vi "predict.vi"(8 "error in (no error)":errorcluster caption="entrée d'erreur (pas d'erreur)", 11 "IsotonicRegression.lvclass 2":refnum<class "IsotonicRegression.lvclass">) -> (0 "error out":errorcluster caption="sortie d'erreur", 2 "C":dbl[][](array[numeric]), 3 "IsotonicRegression.lvclass":refnum<class "IsotonicRegression.lvclass">)   [LabVIEW 2020, in "IsotonicRegression.lvclass"]
doc: "Predict new data by linear interpolation."
uses:
  IsotonicRegression.lvclass
  C:/Users/cipop/TDF Dropbox/2_Technologies de France/1 - Services et Etudes/PLAIY/2 - DEV/PLAIYLAB/code/Python/Python.lvclass
  C:/Users/cipop/TDF Dropbox/2_Technologies de France/1 - Services et Etudes/PLAIY/2 - DEV/PLAIYLAB/code/Model/Model.lvclass
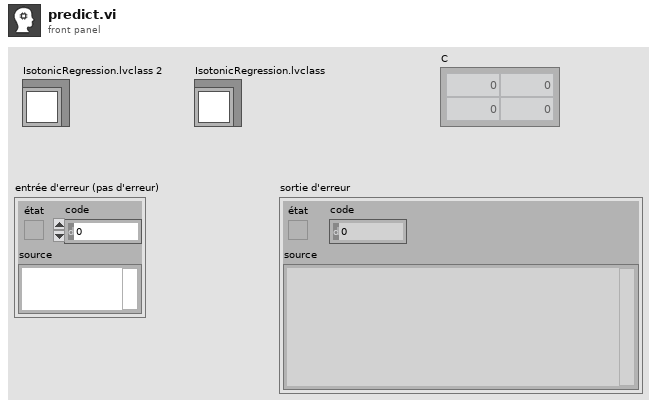
[diagram p1: front panel]
types:
  T1 = typedef "data.ctl" = cluster{"name":string, "X":dbl[][]}
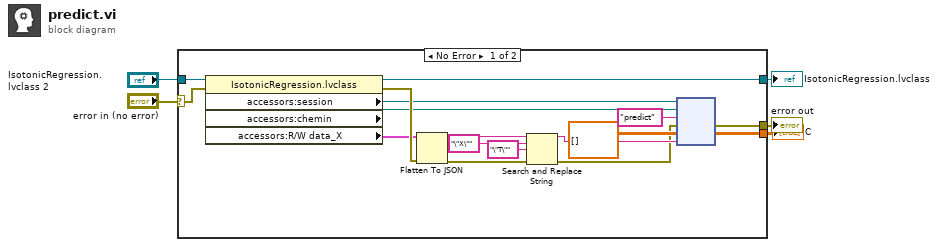
[diagram p0: block diagram]
diagram:
  n1 = case shown="No Error" "error in (no error)" {
    selector: "error in (no error)" -> [w20 w24]
    tunnel: [w21 w24] -> w4
    tunnel: [w15 w23] -> w2
    tunnel: "IsotonicRegression.lvclass 2" -> [w14 w23]
    tunnel: [w12 _] -> w1
    frame No Error {
      n2 = property class="IsotonicRegression.lvclass"(reference=w14, error in=w20) -> (reference out=w15:refnum<class "IsotonicRegression.lvclass">, error out=w19:errorcluster, "accessors:session"=w17:refnum<k35>, "accessors:chemin"=w16:path, "accessors:R/W data_X"=w18:T1)
      n3 = Flatten To JSON(anything=w18, error in (no error)=w19) -> (JSON string=w11:string, 11:w8:errorcluster)  [unwired: 1 in]
      n4 = Search and Replace String(input string=w11, search string="\"X\"", replace string="\"T\"" ("replace string (\"\")"), error in=w8) -> (result string=w7:string, error out=w6:errorcluster)  [unwired: 4 in, 2 out]
      n5 = node(w17, w16, "predict" ("nom de la fonction"), w6, dbl[][] [], w7) -> (w21:errorcluster, w12:dbl[][])  [unwired: 1 in, 3 out]
    }
    frame Error {
    }
  }
  "error out" <- w4
  "IsotonicRegression.lvclass" <- w2
  "C" <- w1
